vi "Search DQMH Module name from selection.vi"(11 "Search Module Name":string="\\Panther Dashboard for DQMH.lvproj\\Coins.lvlib\\Broadcast\\Error Reported") -> (0 "Broadcast?":bool)   [LabVIEW 2020]
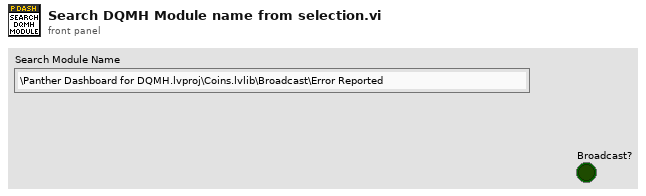
[diagram p1: front panel]
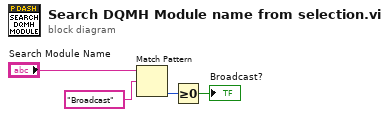
[diagram p0: block diagram]
diagram:
  n1 = Match Pattern(string="Search Module Name", regular expression="Broadcast") -> (offset past match=w2:i32)  [unwired: 1 in, 3 out]
  n2 = Greater Or Equal To 0?(x=w2) -> (x >= 0?=→"Broadcast?":bool)
